vi "Test Child Method.vi"(8 "error in (no error)":errorcluster, 11 "Test Case Test Double Child in":refnum<class "Test Case Test Double Child.lvclass">) -> (0 "error out":errorcluster, 3 "Test Case Test Double Child out":refnum<class "Test Case Test Double Child.lvclass">)   [LabVIEW 2020, in "Test Case Test Double Child.lvclass"]
uses:
  Test Case Test Double Child.lvclass
  C:/Program Files (x86)/National Instruments/LabVIEW 2020/vi.lib/Astemes/LUnit/Test Case.lvclass
  <vilib>/Astemes/LUnit/Test Case.lvclass/Test Case.ctl
  <vilib>/Astemes/LUnit/Append Fail Result.vi
  <vilib>/Astemes/LUnit/Append Pass Result.vi
  <vilib>/Astemes/LUnit/Run In UI.vi
  <vilib>/Utility/error.llb/Clear Errors.vi
  <vilib>/Astemes/LUnit/Test Case.lvclass
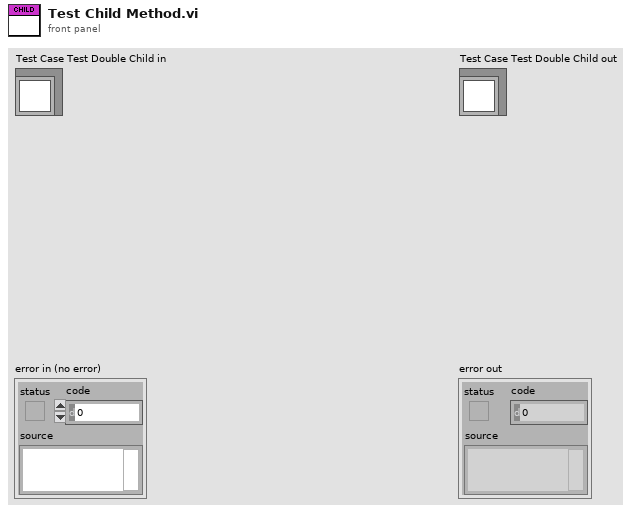
[diagram p1: front panel]
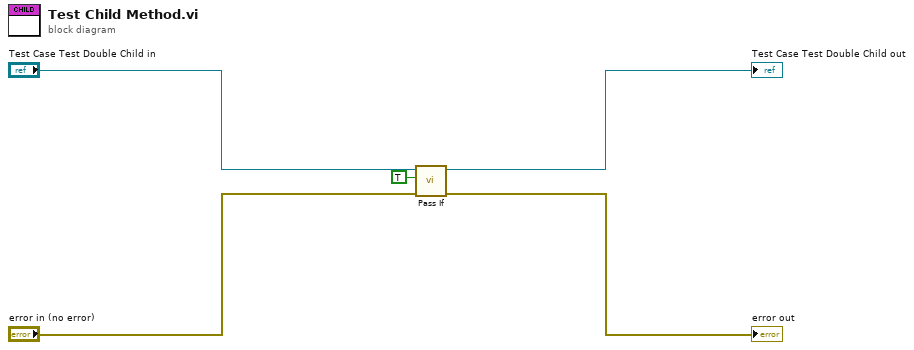
[diagram p0: block diagram]
diagram:
  n1 = call <vilib>:"Pass If.vi"("error in (no error)"="error in (no error)", "Pass?"=TRUE, "LUnit Test Case In"="Test Case Test Double Child in") -> ("error out"=→"error out":errorcluster, "LUnit Test Case Out"=→"Test Case Test Double Child out":refnum<class "Test Case Test Double Child.lvclass">)  [unwired: 7 in]
